vi "EditOptions.vi"(8 "error in":errorcluster, 11 "node in":refnum<class "CI Project.lvclass">) -> (0 "error out":errorcluster, 1 "edit options":T1, 2 "subnodes class":T2, 3 "node out":refnum<class "CI Project.lvclass">)   [LabVIEW 2014, in "CI Project.lvclass"]
doc: "Contains the options for the Menu that will be displayed when doing right click on an item.\nThe sub nodes class configures which nodes can be added to this nodes\nAnd the edit options determine which options are available for the node.\nThis configuration is stored in this VI in case some dynamic configuration is required for the menu options or sub nodes."
uses:
  CI Project.lvclass
  <vilib>/ni/Configuration Framework/Node/SubNodeCluster.ctl
  <vilib>/ni/Configuration Framework/Node/NodeMenuOptions.ctl
  <vilib>/ni/Configuration Framework/class discovery singleton/class discovery singleton methods.ctl
  <vilib>/ni/Configuration Framework/Node/NISE_CEF_Node.lvclass
  <vilib>/ni/Configuration Framework/class discovery singleton/class discovery singleton.lvlib
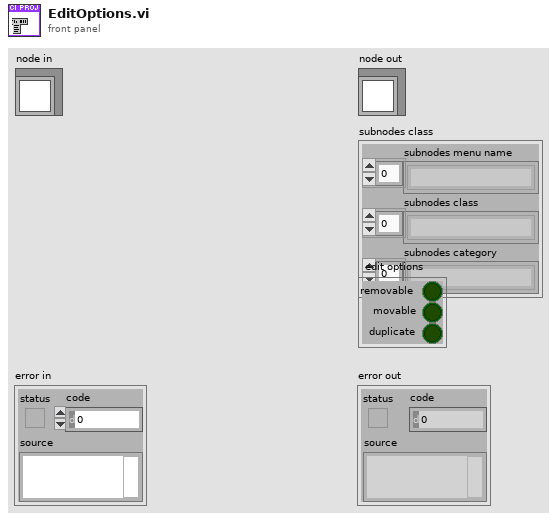
[diagram p1: front panel]
types:
  T1 = typedef "NISE_CEF_Node.lvclass/NodeMenuOptions.ctl" = cluster{"removable":bool, "movable":bool, "duplicate":bool}
  T2 = typedef "NISE_CEF_Node.lvclass/SubNodeCluster.ctl" = cluster{"subnodes menu name":string[], "subnodes class":string[], "subnodes category":string[]}
  T3 = typedef "class discovery singleton.lvlib/class discovery singleton methods.ctl" = enum16{"add search paths", "load class by name", "list available classes", "get class path", "delete cache"}
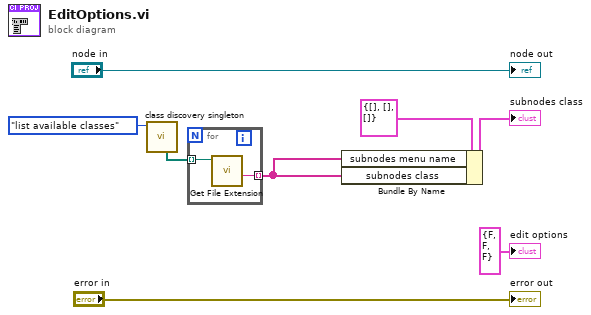
[diagram p0: block diagram]
diagram:
  n1 = call <vilib>:"class discovery singleton.vi"("method"=class_discovery_singleton_methods."list available classes") -> ("discovered classes"=w2:path[])  [unwired: 7 in, 3 out]
  n2 = for {
    tunnel: w2 -> [w10] mode=indexing
    tunnel: [w9] -> w1 mode=indexing
    n3 = call <vilib>:"Get File Extension.vi"("file"=w10) -> ("filename without extension"=w9:string)  [unwired: 7 in, 3 out]
  }
  n4 = Bundle By Name(cluster=T2 {"subnodes menu name"=[], "subnodes class"=[], "subnodes category"=[]} ("subnodes class"), "subnodes menu name"=w1, "subnodes class"=w1) -> (→"subnodes class":T2)
  "error out" <- "error in"
  "node out" <- "node in"
  "edit options" <- T1 {"removable"=FALSE, "movable"=FALSE, "duplicate"=FALSE} ("edit options")
